vi "Robot Info Loop.vi"   [LabVIEW 2017]
uses:
  Robot Global Data.vi
types:
  T1 = typedef "WPI_DriverStationRobotMode2.ctl" = enum16{"Autonomous Disabled", "Autonomous Enabled", "Teleop Disabled", "Teleop Enabled", "Disconnected", "Finish", "Test Disabled", "Test Enabled", "Emergency Stopped"}
  T2 = typedef "WPI_DriverStationPositionInfo.ctl" = enum16{"1", "2", "3"}
  T3 = typedef "WPI_DriverStationAllianceInfo.ctl" = enum16{"Red", "Blue", "Invalid"}
  T4 = typedef "Robot Info.ctl" = cluster{"FMS":bool, "Switch and Scale Sides":string, "Event Name":string, "Alliance":T3, "Position":T2, "Match Number":u16, "Robot Mode":T1, "Match Time(s)":sgl}
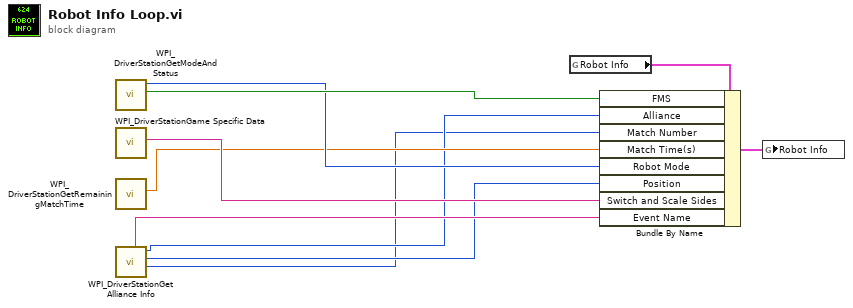
[diagram p0: block diagram]
diagram:
  n1 = call <vilib>:"WPI_DriverStationGetModeAndStatus.vi"() -> ("FMS Attached"=w8:bool, "Robot Mode"=w7:T1)  [unwired: 10 in]
  n2 = call <vilib>:"WPI_DriverStationGame Specific Data.vi"() -> ("Game Specific Data"=w6:string)  [unwired: 11 in]
  n3 = call <vilib>:"WPI_DriverStationGetRemainingMatchTime.vi"() -> ("Match Time(s)"=w5:sgl)  [unwired: 10 in, 1 out]
  n4 = call <vilib>:"WPI_DriverStationGet Alliance Info.vi"() -> ("Match Number"=w1:u16, "Position"=w2:T2, "Alliance"=w3:T3, "Event Name"=w4:string)  [unwired: 6 in, 2 out]
  n5 = global read "Robot Global Data.vi" "Robot Info"() -> (w10:T4)
  n6 = Bundle By Name(cluster=w10, "FMS"=w8, "Alliance"=w3, "Match Number"=w1, "Match Time(s)"=w5, "Robot Mode"=w7, "Position"=w2, "Switch and Scale Sides"=w6, "Event Name"=w4) -> (w9:T4)
  n7 = global write "Robot Global Data.vi" "Robot Info"(w9) -> ()
